vi "Actor Core.vi"(8 "error in":errorcluster, 11 "Connection Handler in":refnum<class "Connection Handler.lvclass">) -> (0 "error out":errorcluster, 3 "Actor out":refnum<class "Actor.lvclass">)   [LabVIEW 2017, in "Connection Handler.lvlib" / "Connection Handler.lvclass"]
doc: "(<B>Filename</B>: Actor Framework.lvlib:Actor.lvclass:Actor Core.vi)\n\nReceives messages to the actor, reacts to them, and initiates any error handling that may shut the actor down.\n\nDescendant classes may override this VI to append parallel tasks for the actor to complete while it handles messages. Overrides use the Call Parent Method node."
uses:
  Connection Handler.lvclass
  <vilib>/ActorFramework/Actor/Actor.lvclass
  Connection Handler.lvclass/Connection Handler.ctl
  Actor wHelper/Actor wHelper/Actor wHelper.lvclass
panel:
  out "ID":i32
  # "Headless Connection Handler"
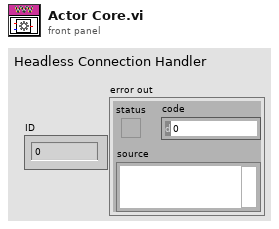
[diagram p1: front panel]
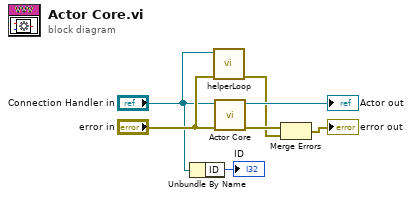
[diagram p0: block diagram]
diagram:
  n1 = Unbundle By Name("Connection Handler in") -> ("ID"=→"ID":i32)
  n2 = call-dynamic "helperLoop.vi"("error in (no error)"="error in", "Connection Handler in"="Connection Handler in") -> ("error out"=w3:errorcluster)  [unwired: 8 in, 1 out]
  n3 = call-parent "Actor Core.vi"("error in"="error in", "Actor in"="Connection Handler in") -> ("error out"=w7:errorcluster, "Actor out"=→"Actor out":refnum<class "Actor.lvclass">)  [unwired: 8 in]
  n4 = Merge Errors(w7, w3) -> (→"error out":errorcluster)
